vi "FGV Initialize.vi"() -> (3 "found?":bool)   [LabVIEW 2020, in "SimpleDependencyInspector.lvlib"]
uses:
  SimpleDependencyInspector.lvlib
  FGV Functions--enum.ctl
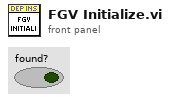
[diagram p1: front panel]
types:
  T1 = typedef "SimpleDependencyInspector.lvlib/FGV Functions--enum.ctl" = enum16{"Initialize", "Get Node ID", "Set Node ID"}
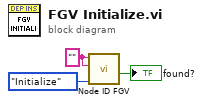
[diagram p0: block diagram]
diagram:
  w1 = "" ("Node ID")
  n1 = call "Node ID FGV.vi"("Initialize"=FGV_Functions--enum."Initialize", "Node Name"=w1, "Node ID"=w1) -> ("found?"=→"found?":bool)  [unwired: 6 in, 2 out]
